vi "Send Close.vi"(8 "error in (no error)":errorcluster, 11 "WebSocket Client in":refnum<class "WebSocket Client.lvclass">) -> (0 "error out":errorcluster, 3 "WebSocket Client out":refnum<class "WebSocket Client.lvclass">)   [LabVIEW 2020, in "HTTP Server.lvlib" / "WebSocket Client.lvclass"]
uses:
  WebSocket Client.lvclass
  WebSocket Client.lvclass/WebSocket Client.ctl
  OpCode.ctl
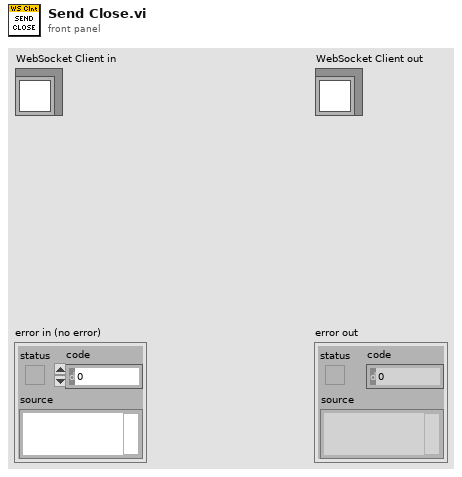
[diagram p1: front panel]
types:
  T1 = typedef "HTTP Server.lvlib/WebSocket Client.lvclass/OpCode.ctl" = enum8{"Continuation", "Text", "Binary", "Reserved3", "Reserved4", "Reserved5", "Reserved6", "Reserved7", "Close", "Ping", "Pong", "ReservedB", "ReservedC", "ReservedD", "ReservedE", "ReservedF"}
  T2 = typedef "HTTP Server.lvlib/WebSocket Client.lvclass/Ref Data.ctl" = cluster{"Closing":bool}
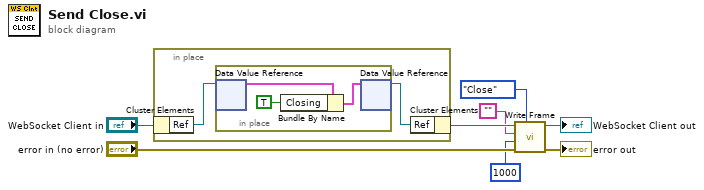
[diagram p0: block diagram]
diagram:
  n1 = in-place {
    n2 = in-place-cluster #1("WebSocket Client in") -> ("Ref"=w10:refnum<data-value>)
    n3 = in-place {
      n4 = in-place-dvr #2(w10) -> (w13:T2)  [unwired: 1 out]
      n5 = Bundle By Name(cluster=w13, "Closing"=TRUE) -> (w11:T2)
      n6 = in-place-dvr #2(w11) -> (w9:refnum<data-value>)  [unwired: 1 out]
    }
    n7 = in-place-cluster #1("Ref"=w9) -> (w5:refnum<class "WebSocket Client.lvclass">)
  }
  n8 = call "Write Frame.vi"("OpCode"=OpCode."Close", "error in (no error)"="error in (no error)", "Timeout ms"=1000, "Payload"="", "WebSocket Client in"=w5) -> ("error out"=→"error out":errorcluster, "WebSocket Client out"=→"WebSocket Client out":refnum<class "WebSocket Client.lvclass">)  [unwired: 4 in, 1 out]
